vi "Arm Angle to Pot Value.vi"(1 "angleInDegrees":dbl, 2 "potValueForArmAtZeroDegrees (pot value)":dbl) -> (0 "Pot Value":sgl)   [LabVIEW 2017]
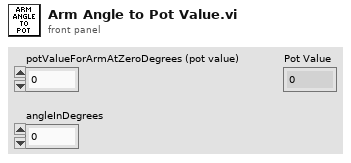
[diagram p1: front panel]
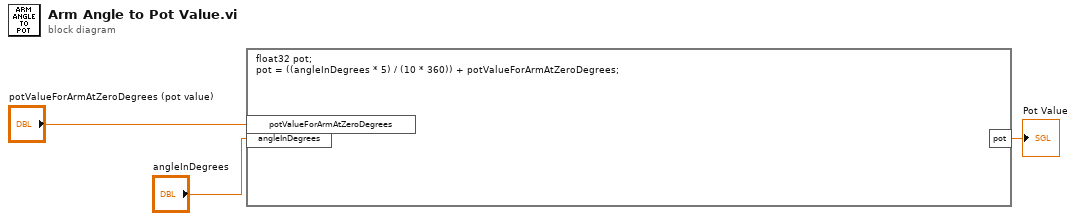
[diagram p0: block diagram]
diagram:
  n1 = formula code="float32 pot;\npot = ((angleInDegrees * 5) / (10 * 360)) + potValueForArmAtZeroDegrees;"("angleInDegrees"="angleInDegrees", "potValueForArmAtZeroDegrees"="potValueForArmAtZeroDegrees (pot value)") -> ("pot"=→"Pot Value":sgl)
